vi "System Function Call Translator If Exists.vi"(8 "Error In":errorcluster, 11 "Node Refnum":refnum<vi>) -> (0 "Error Out":errorcluster, 1 "Defines":string[](array[string]), 2 "Includes":string[](array[string])=["<Arduino.h>", "<math.h>"], 3 "Replaced Code":string="a = floor(v);")   [LabVIEW 2014]
doc: "Run Translator.vi if it's there in same directory as SubVI. If SubVI refnum not providedd it's using VI path control."
panel:
  in  "Output Datatypes":string[](array[string])=["int"]
  in  "Input Datatypes":string[](array[string])=["error", "int"]
  in  "Outputs":string[](array[string])=["a"]
  in  "Inputs":string[](array[string])=["error in", "x"]
  in  "Function Name":string="Arduino Math.lvlib:Floor"
  # "JUST FOR NOW, DEBUGGING"
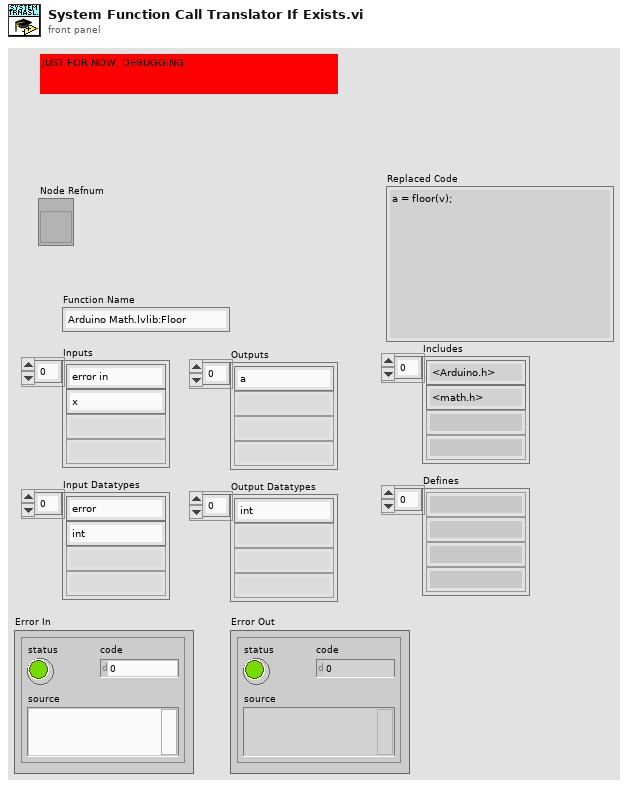
[diagram p1: front panel]
types:
  T1 = cluster{"terminals datatypes":string[][], "terminal\nconnected?":bool[], "terminal captions":string[], "term. count":i32, "terminal\nIsSource?":bool[], "SubVI name":string, "connected\nwires refs.":refnum<vi>[], "coerced dot?":bool[], "terminals[]":refnum<vi>[]}
  T2 = cluster{"wire labels":string[], "wire terminals datatypes":string[][]}
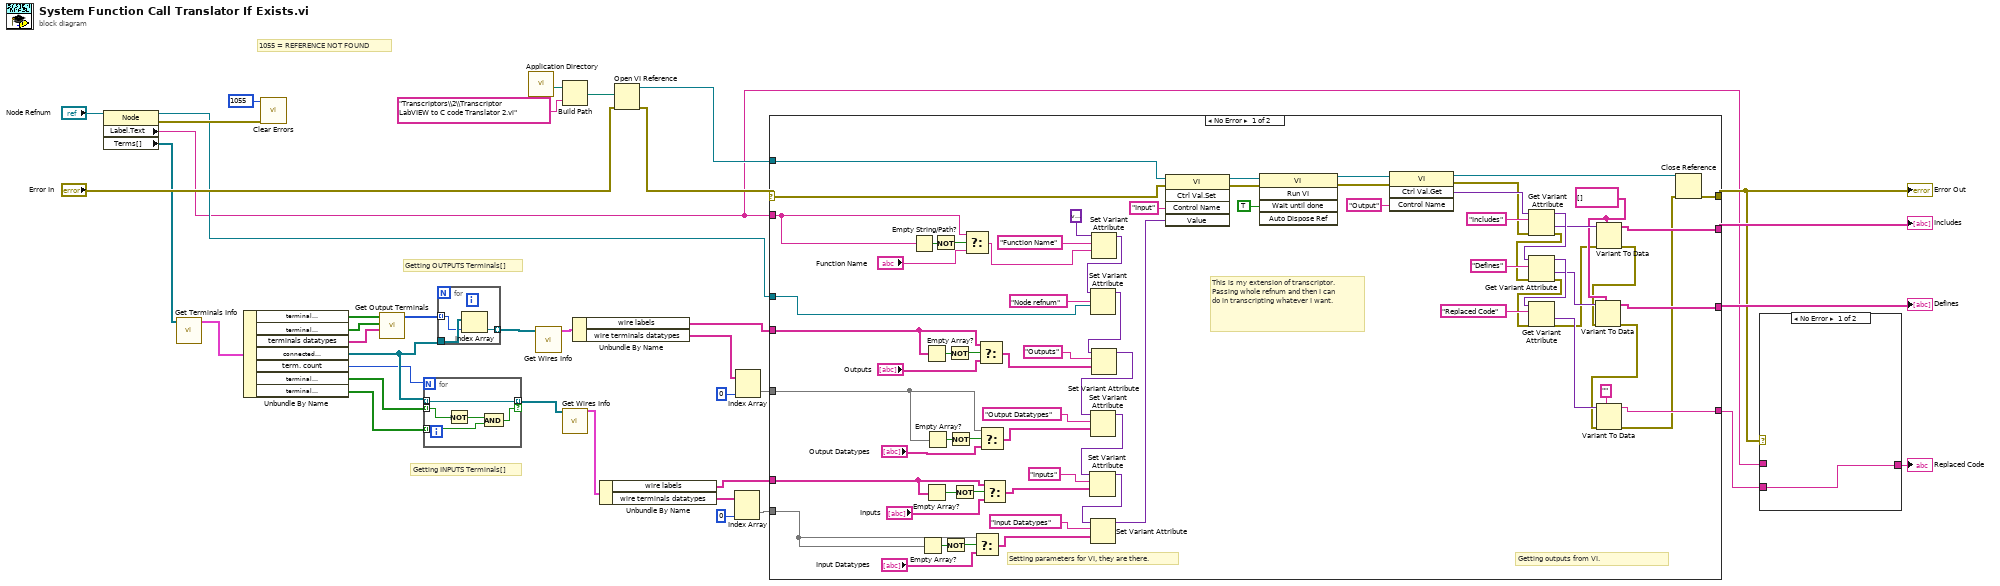
[diagram p0: block diagram]
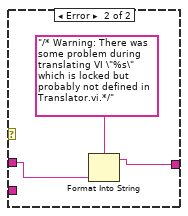
[diagram p2: hidden frame]
diagram:
  # "Getting INPUTS Terminals[]"
  # "Getting OUTPUTS Terminals[]"
  # "1055 = REFERENCE NOT FOUND"
  n1 = property class="Node"(reference="Node Refnum") -> (reference out=w7:refnum<vi>, error out=w35:errorcluster, "Label.Text"=w2:string, "Terms[]"=w3:refnum<vi>[])  [unwired: 1 in]
  n2 = call "Get Terminals Info.vi"("Terms[]"=w3) -> ("output cluster"=w33:T1)  [unwired: 9 in, 1 out]
  n3 = Unbundle By Name(w33) -> ("terminal\nconnected?"=w32:bool[], "terminal\nIsSource?"=w31:bool[], "terminals datatypes"=w30:string[][], "connected\nwires refs."=w23:refnum<vi>[], "term. count"=w22:i32, "terminal\nIsSource?"=w13:bool[], "terminal\nconnected?"=w12:bool[])
  n4 = call <vilib>:"Clear Errors.vi"("error in (no error)"=w35, "specific error code to clear (0: all)"=1055) -> ()  [unwired: 4 in, 2 out]
  n5 = call "Get Output Terminals.vi"("terminals datatypes"=w30, "isSource?"=w31, "isConnected?"=w32) -> ("output terminals indexes"=w21:i32[])  [unwired: 8 in]
  n6 = for {
    N: w22 -> [_]
    tunnel: w23 -> [w42] mode=indexing
    tunnel: w13 -> [w43] mode=indexing
    tunnel: [w42] -> w11 mode=indexing if=w39
    tunnel: w12 -> [w40] mode=indexing
    n7 = Not(x=w43) -> (.not. x?=w41:bool)
    n8 = And(x=w41, y=w40) -> (x .and. y?=w39:bool)
  }
  n9 = for {
    tunnel: w21 -> [w45] mode=indexing
    tunnel: w23 -> [w46]
    tunnel: [w44] -> w29 mode=indexing
    n10 = Index Array(array=w46, index=w45) -> (element=w44:refnum<vi>)
  }
  n11 = call <vilib>:"Application Directory.vi"() -> ("Application Directory"=w5:path)
  n12 = call "Get Wires Info.vi"("connected\nwires refs."=w29) -> ("output cluster 2"=w28:T2)  [unwired: 10 in]
  n13 = Build Path(base path=w5, name or relative path="Transcriptors\\2\\Transcriptor LabVIEW to C code Translator 2.vi") -> (appended path=w4:path)
  n14 = call "Get Wires Info.vi"("connected\nwires refs."=w11) -> ("output cluster 2"=w20:T2)  [unwired: 10 in]
  n15 = Unbundle By Name(w28) -> ("wire labels"=w27:string[], "wire terminals datatypes"=w26:string[][])
  n16 = Unbundle By Name(w20) -> ("wire labels"=w16:string[], "wire terminals datatypes"=w18:string[][])
  n17 = Open VI Reference(vi path=w4, error in (no error)="Error In") -> (vi reference=w10:refnum<vi>, error out=w8:errorcluster)  [unwired: 4 in]
  n18 = Index Array(array=w18, index (col)=0 ("disabled index (col)")) -> (element=w17:string[])  [unwired: 1 in]
  n19 = Index Array(array=w26, index (col)=0 ("disabled index (col)")) -> (element=w24:string[])  [unwired: 1 in]
  n20 = case shown="No Error" w8 {
    selector: w8 -> [w52 w118]
    tunnel: [w117 w118] -> w15
    tunnel: [w90 _] -> w38
    tunnel: [w89 _] -> w37
    tunnel: [w88 _] -> w1
    tunnel: w27 -> [w81 _]
    tunnel: w24 -> [w68 _]
    tunnel: w17 -> [w69 _]
    tunnel: w16 -> [w61 _]
    tunnel: w10 -> [w53 _]
    tunnel: w7 -> [w48 _]
    tunnel: w2 -> [w47 _]
    frame No Error {
      w92 = string[] [] ("Array - String")
      # "This is my extension of transcriptor. Passing whole refnum and then I can do in transcripting whatever I want."
      # "Getting outputs from VI."
      # "Setting parameters for VI, they are there."
      n21 = Empty String/Path?(string/path=w47) -> (empty?=w87:bool)
      n22 = Empty Array?(array=w69) -> (empty?=w75:bool)
      n23 = Empty Array?(array=w81) -> (empty?=w80:bool)
      n24 = Empty Array?(array=w61) -> (empty?=w62:bool)
      n25 = Empty Array?(array=w68) -> (empty?=w76:bool)
      n26 = Not(x=w87) -> (.not. x?=w86:bool)
      n27 = Not(x=w75) -> (.not. x?=w74:bool)
      n28 = Not(x=w80) -> (.not. x?=w79:bool)
      n29 = Not(x=w76) -> (.not. x?=w77:bool)
      n30 = Not(x=w62) -> (.not. x?=w63:bool)
      n31 = Select(t=w47, s=w86, f="Function Name") -> (s? t:f=w85:string)
      n32 = Select(t=w69, s=w74, f="Input Datatypes") -> (s? t:f=w73:string[])
      n33 = Select(t=w81, s=w79, f="Outputs") -> (s? t:f=w78:string[])
      n34 = Select(t=w68, s=w77, f="Output Datatypes") -> (s? t:f=w72:string[])
      n35 = Select(t=w61, s=w63, f="Inputs") -> (s? t:f=w65:string[])
      n36 = Set Variant Attribute(Variant=variant ("Value"), name="Function Name", value=w85) -> (Variant out=w51:variant)  [unwired: 1 in, 2 out]
      n37 = Set Variant Attribute(Variant=w51, name="Node refnum", value=w48) -> (Variant out=w50:variant)  [unwired: 1 in, 2 out]
      n38 = Set Variant Attribute(Variant=w50, name="Outputs", value=w78) -> (Variant out=w110:variant)  [unwired: 1 in, 2 out]
      n39 = Set Variant Attribute(Variant=w110, name="Output Datatypes", value=w72) -> (Variant out=w67:variant)  [unwired: 1 in, 2 out]
      n40 = Set Variant Attribute(Variant=w67, name="Inputs", value=w65) -> (Variant out=w66:variant)  [unwired: 1 in, 2 out]
      n41 = Set Variant Attribute(Variant=w66, name="Input Datatypes", value=w73) -> (Variant out=w108:variant)  [unwired: 1 in, 2 out]
      n42 = invoke class="VI" method="Ctrl Val.Set"(reference=w53, error in=w52, "Control Name"="Input", "Value"=w108) -> (reference out=w104:refnum<vi>, error out=w103:errorcluster)  [unwired: 1 in, 3 out]
      n43 = invoke class="VI" method="Run VI"(reference=w104, error in=w103, "Wait until done"=TRUE ("Wait Until Done")) -> (reference out=w107:refnum<vi>, error out=w106:errorcluster)  [unwired: 2 in, 3 out]
      n44 = invoke class="VI" method="Ctrl Val.Get"(reference=w107, error in=w106, "Control Name"="Output") -> (reference out=w101:refnum<vi>, error out=w60:errorcluster, "Get Control Value Variant"=w102:variant)  [unwired: 1 in, 1 out]
      n45 = Get Variant Attribute(Variant=w102, name="Includes", error in=w60) -> (duplicate Variant=w97:variant, value=w95:variant, error out=w59:errorcluster)  [unwired: 1 in, 1 out]
      n46 = Get Variant Attribute(Variant=w97, name="Defines", error in=w59) -> (duplicate Variant=w96:variant, value=w94:variant, error out=w58:errorcluster)  [unwired: 1 in, 1 out]
      n47 = Get Variant Attribute(Variant=w96, name="Replaced Code", error in=w58) -> (value=w93:variant, error out=w57:errorcluster)  [unwired: 1 in, 2 out]
      n48 = Variant To Data(error in=w57, type=w92, Variant=w95) -> (data=w90:string[], error out=w56:errorcluster)
      n49 = Variant To Data(error in=w56, type=w92, Variant=w94) -> (data=w89:string[], error out=w55:errorcluster)
      n50 = Variant To Data(error in=w55, type="" ("name"), Variant=w93) -> (data=w88:string, error out=w54:errorcluster)
      n51 = Close Reference(reference=w101, error in (no error)=w54) -> (error out=w117:errorcluster)
    }
    frame Error {
    }
  }
  "Error Out" <- w15
  "Includes" <- w38
  "Defines" <- w37
  n52 = case shown="No Error" w15 {
    tunnel: [w119 w121] -> w14
    tunnel: w2 -> [_ w120]
    tunnel: w1 -> [w119 _]
    frame No Error {
    }
    frame Error {
      n53 = Format Into String(format string="/* Warning: There was some problem during translating VI \"%s\" which is locked but probably not defined in Translator.vi.*/", w120) -> (resulting string=w121:string)  [unwired: 2 in, 1 out]
    }
  }
  "Replaced Code" <- w14
